vi "JSON Example.vi"() -> ()   [LabVIEW 2015]
uses:
  lib/JSON.lvlib
panel:
  out "Parsed Data":T1
  out "JSON String":string
  in  "Tree":string(tree)
  in  "JSON String":string="# This is a TOML document.\n\ntitle = \"TOML Example\"\n\n[owner]\nname = \"David Taylor\"\ndob = 1991-07-17T07:12:00-07:00 # First class dates\n\n[database]\nserver = \"192.168.1.1\"\nports = [ 8001, 8001, 8002 ]\nconnection_max = 5000\nenabled = true\n\n[servers]\n\n  # Indentation (tabs and/or spaces) is allowed but not required\n  [servers.alpha]\n  ip = \"10.0.0.1\"\n  dc = \"eqdc10\"\n\n  [servers.beta]\n  ip = \"10.0.0.2\"\n  dc = \"eqdc10\"\n\n[clients]\ndata = [ [\"gamma\", \"delta\"], [1, 2] ]\n\n# Line breaks are OK when inside arrays\nhosts = [\n  \"alpha\",\n  \"omega\"\n]\n\n#inline table\ninline_table = {one = 1, two = 2}\n\n[[array_of_tables]]\nmulti-line-string = \"\"\"\nline one\nline two\"\"\"\n\n[[array_of_tables]]\nmulti-line-literal-string = '''\nliteral strings allow special characters \\ unescaped\nline two'''"
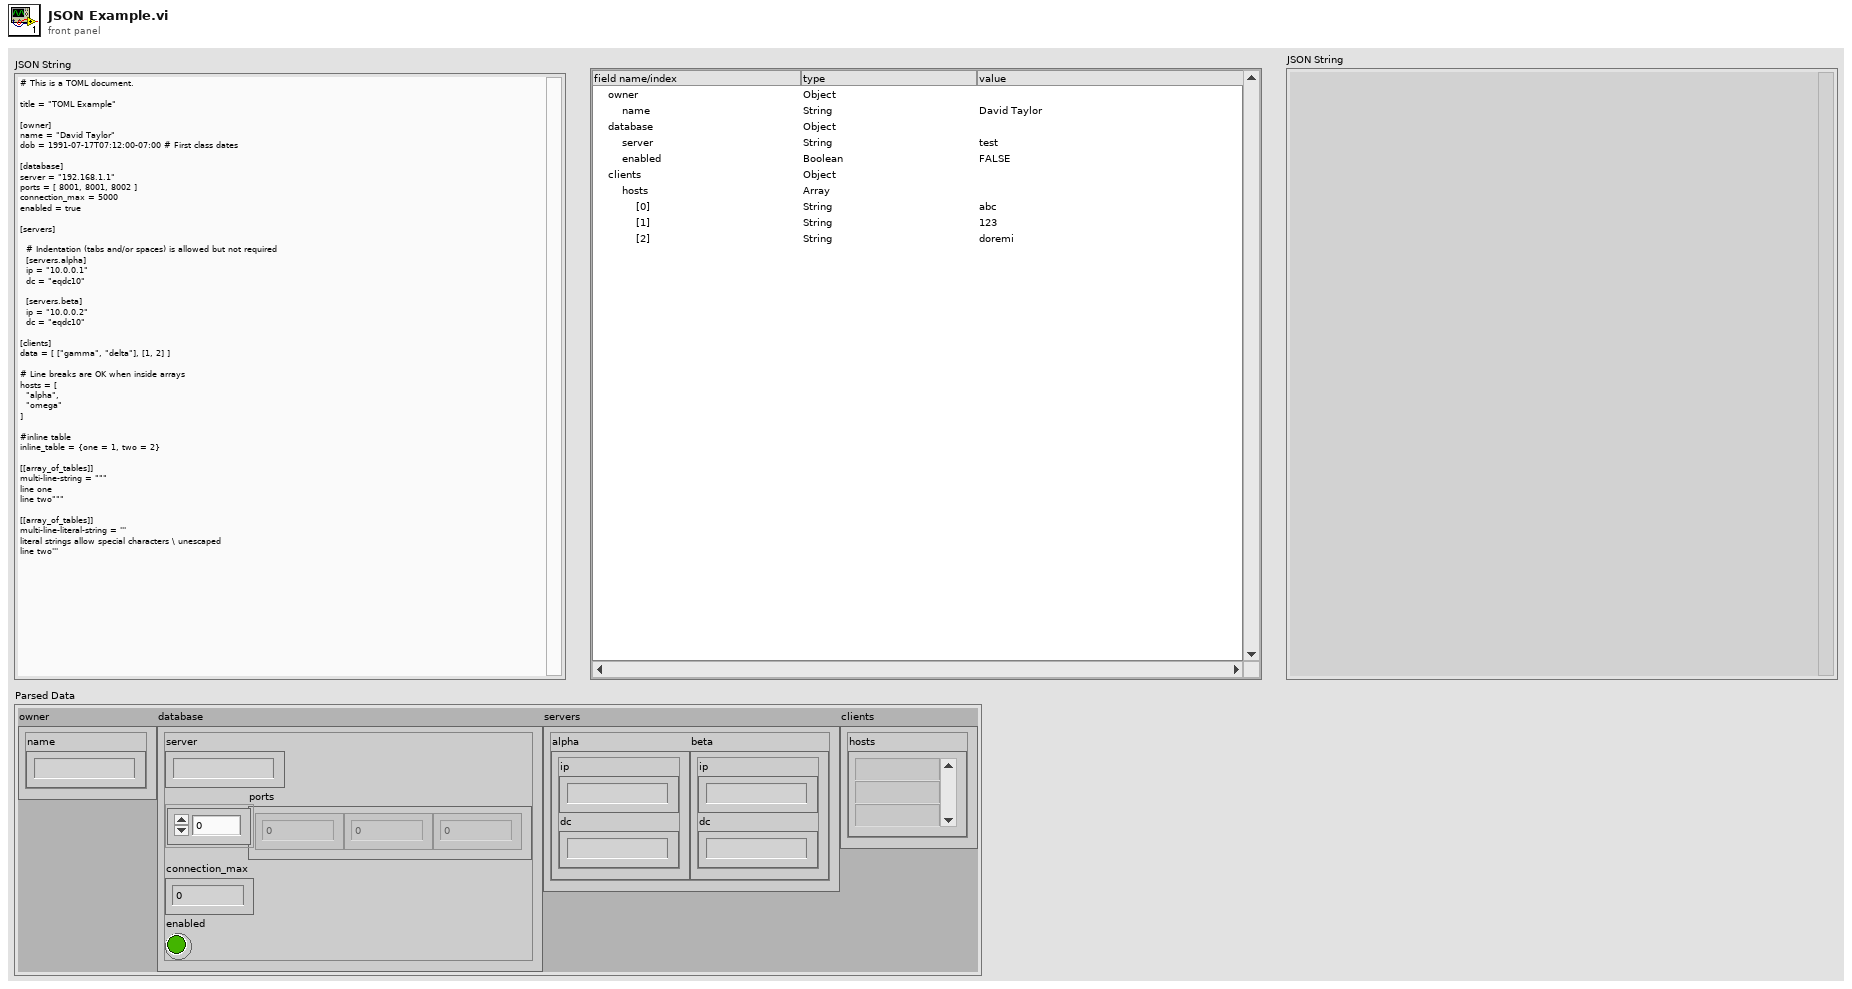
[diagram p1: front panel]
types:
  T1 = cluster{"owner":cluster{"name":string}, "database":cluster{"server":string, "ports":dbl[], "connection_max":dbl, "enabled":bool}, "servers":cluster{"alpha":cluster{"ip":string, "dc":string}, "beta":cluster{"ip":string, "dc":string}}, "clients":cluster{"hosts":string[]}}
  T2 = typedef "JSON.lvlib/JSON Value.ctl" = cluster{"\\type":enum16{"Object", "Array", "String", "Number", "Boolean", "Null"}, "ÿýÿýÿýÿýÿýÿþÿýÿýÿý&LV-JSON.lvlib:JSON Name-Value Pair.ctlÿýÿýÿýÿýÿýÿþÿýÿýÿýLV-JSON.lvlib:JSON Value.ctl":variant}
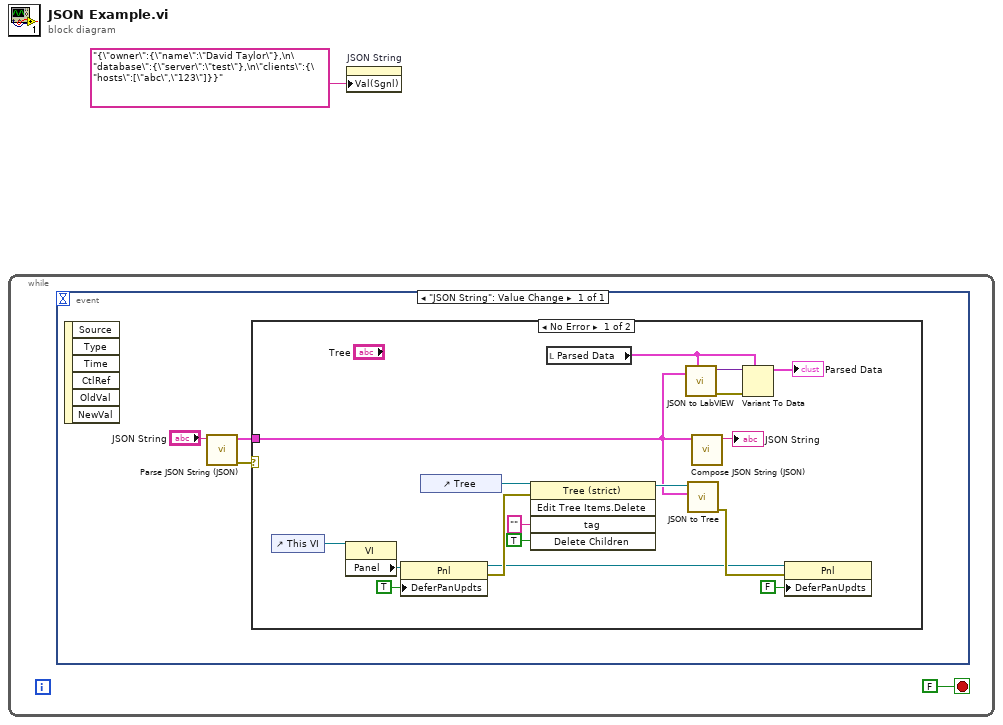
[diagram p0: block diagram]
diagram:
  n1 = while {
    stop <- FALSE stop-if-true
    n2 = event shown="[0] \"JSON String\": Value Change" {
      selector: _ -> [_]
      dyn-events: _ -> [_]
      timeout: _ -> [_]
      event "JSON String": Value Change {
        n3 = event-data() -> ()  [unwired: 1 in, 6 out]
        n4 = call "Parse JSON String (JSON).vi"("String"="JSON String") -> ("error out"=w5:errorcluster, "Value"=w3:T2)  [unwired: 9 in]
        n5 = case shown="No Error" w5 {
          tunnel: w3 -> [w8 _]
          frame No Error {
            n6 = control-ref of="This VI"() -> (w18:refnum<vi>)
            n7 = property class="VI"(reference=w18) -> ("Panel"=w17:refnum<vi>)  [unwired: 1 in, 2 out]
            n8 = property class="Pnl"(reference=w17, "DeferPanUpdts"=TRUE ("Defer Panel Updates")) -> (reference out=w13:refnum<vi>, error out=w15:errorcluster)  [unwired: 1 in]
            n9 = control-ref of="Tree"() -> (w22:refnum<vi>)
            n10 = invoke class="Tree (strict)" method="Edit Tree Items.Delete"(reference=w22, error in=w15, "tag"="" ("Tag"), "Delete Children"=TRUE ("Delete Children?")) -> (reference out=w19:refnum<vi>)  [unwired: 1 in, 4 out]
            n11 = local read "Parsed Data"() -> (w10:T1)
            n12 = call "JSON to LabVIEW.vi"("Default Value"=w10, "JSON Value"=w8) -> ("error out"=w6:errorcluster, "LV Value"=w7:variant)  [unwired: 8 in]
            n13 = call "JSON to Tree.vi"("Value"=w8, "TreeControl in"=w19) -> ("error out"=w14:errorcluster)  [unwired: 9 in]
            n14 = call "Compose JSON String (JSON).vi"("Value"=w8) -> ("String"=→"JSON String":string)  [unwired: 9 in, 1 out]
            n15 = Variant To Data(error in=w6, type=w10, Variant=w7) -> (data=→"Parsed Data":T1)  [unwired: 1 out]
            n16 = property class="Pnl"(reference=w13, error in=w14, "DeferPanUpdts"=FALSE ("Defer Panel Updates")) -> ()  [unwired: 2 out]
          }
          frame Error {
          }
        }
      }
    }
  }
  n17 = property on="JSON String" class="Str"("Val(Sgnl)"="{\"owner\":{\"name\":\"David Taylor\"},\n\"database\":{\"server\":\"test\"},\n\"clients\":{\"hosts\":[\"abc\",\"123\"]}}" ("TOML String")) -> ()  [unwired: 2 in, 2 out]
